vi "Image Display Controller-subvi.vi"() -> ()   [LabVIEW 2014]
doc: "This widget allows the user to separately adjust the properties of mulltiple, independently displayed image windows. The controller is a stand-alone VI that can run in a separate thread from the program that is producing the images, so that the image display settings can be adjusted whilst other things (e.g., data acquisition) are occurring simultaneously."
uses:
  ctt's/Image to Display event.ctt
  <vilib>/vision/Image Controls.llb/IMAQ Image.ctl
  Globals/Initilize Globals.vi
panel:
  in  "Presets":T1(array[cluster])=[{"Mem"=FALSE, "Black"=-32500.0, "White"=-25000.0, "Recall"=FALSE}]
  in  "Keep this in corner?":bool=TRUE
  in  "Autosize M":bool
  in  "Autoposition M":bool
  in  "Autoscale M":bool
  in  "Zoom +":bool
  in  "Zoom -":bool
  out "In use":bool
  in  "Auto size":bool
  in  "Auto position":bool
  in  "Autoscale":bool
  out "Window Title":string
  in  "Control image window #":u8(slide)=1 max=1 step=1 scale=0.0..1.0
  out "error out":errorcluster
  out "Black/White Levels temp":cluster{ext, ext}(slide)={1.0, 65535.0} scale=-32767.0..327567.0
  in  "Black/White Levels":cluster{ext, ext}(slide)={1.0, 65535.0} scale=-32767.0..327567.0
  in  "Stop":bool
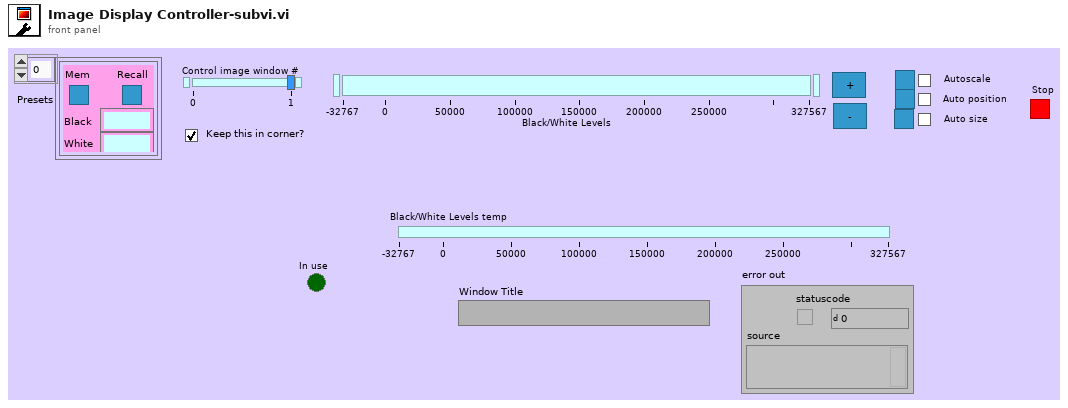
[diagram p1: front panel]
types:
  T1 = cluster{"Mem":bool, "Black":ext, "White":ext, "Recall":bool}[]
  T2 = typedef "Image Type" = u32
  T3 = typedef "IMAQ Image.ctl" = refnum<image>
  T4 = cluster{"Image Type":T2, "Image":T3, "Initialized?":bool, "Window Title":string, "Auto resize?":bool, "Auto position?":bool, "Autoscale?":bool, "Black/White Levels":cluster{ext, ext}, "Scale Min":ext, "Scale Max":ext}
  T5 = typedef "LVRectTypeDef.ctl" = cluster{"Left":i16, "Top":i16, "Right":i16, "Bottom":i16}
  T6 = typedef "Image to Display event.ctt" = cluster{"Image":T3, "Window Title":string, "Window Number":i32, "Image Type":T2, "Quit display controller?":bool}
  T7 = cluster{"Image Type":T2, "Image":T3, "Initialized?":bool, "Window Title":string, "Auto resize?":bool, "Auto position?":bool, "Autoscale?":bool, "Black/White Levels":cluster{ext, ext}, "Scale Min":ext, "Scale Max":ext}[]
  T8 = cluster{"Mem":bool, "Black":ext, "White":ext, "Recall":bool}
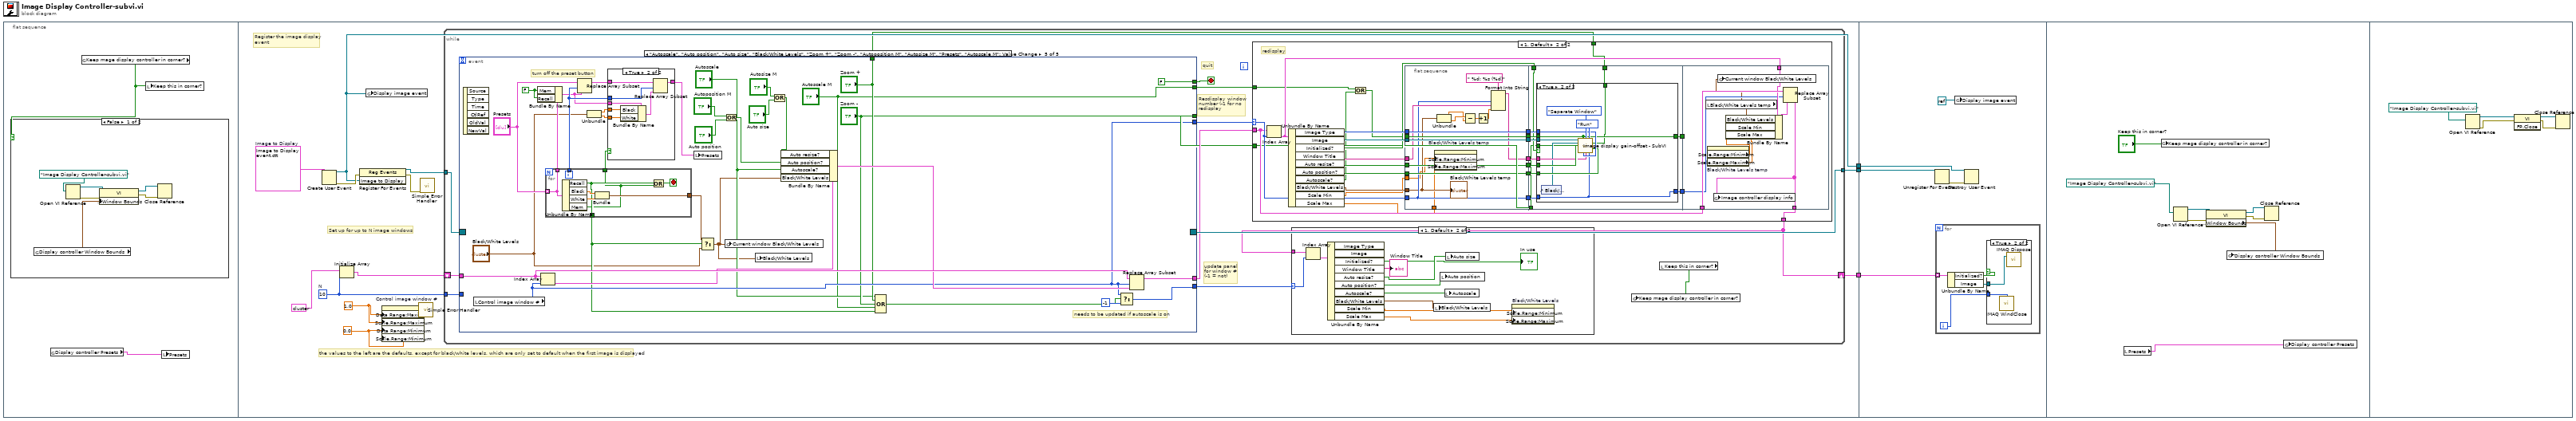
[diagram p0: block diagram]
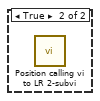
[diagram p2: hidden frame]
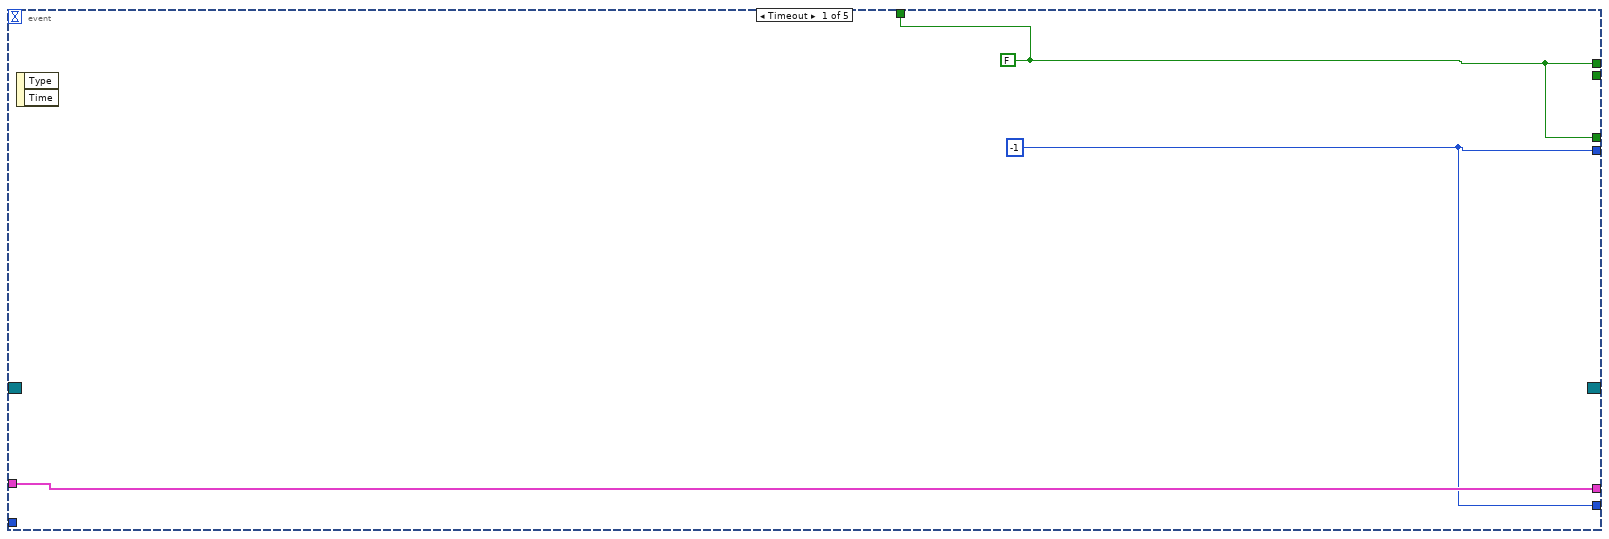
[diagram p6: hidden frame]
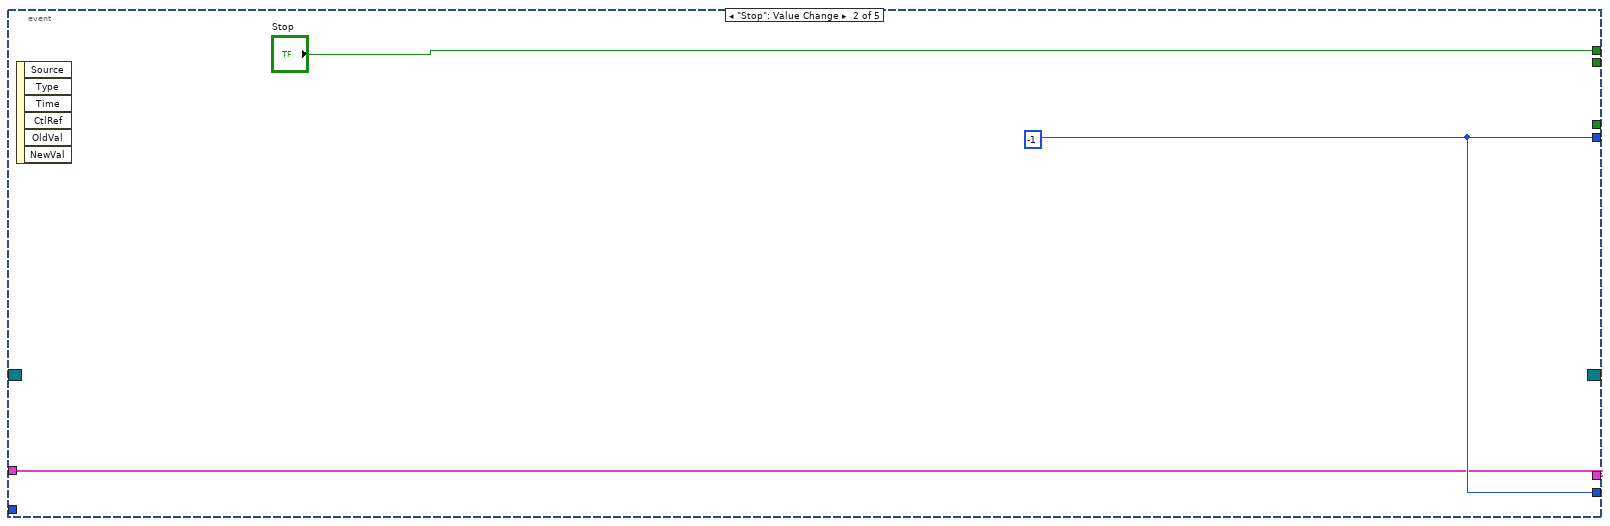
[diagram p7: hidden frame]
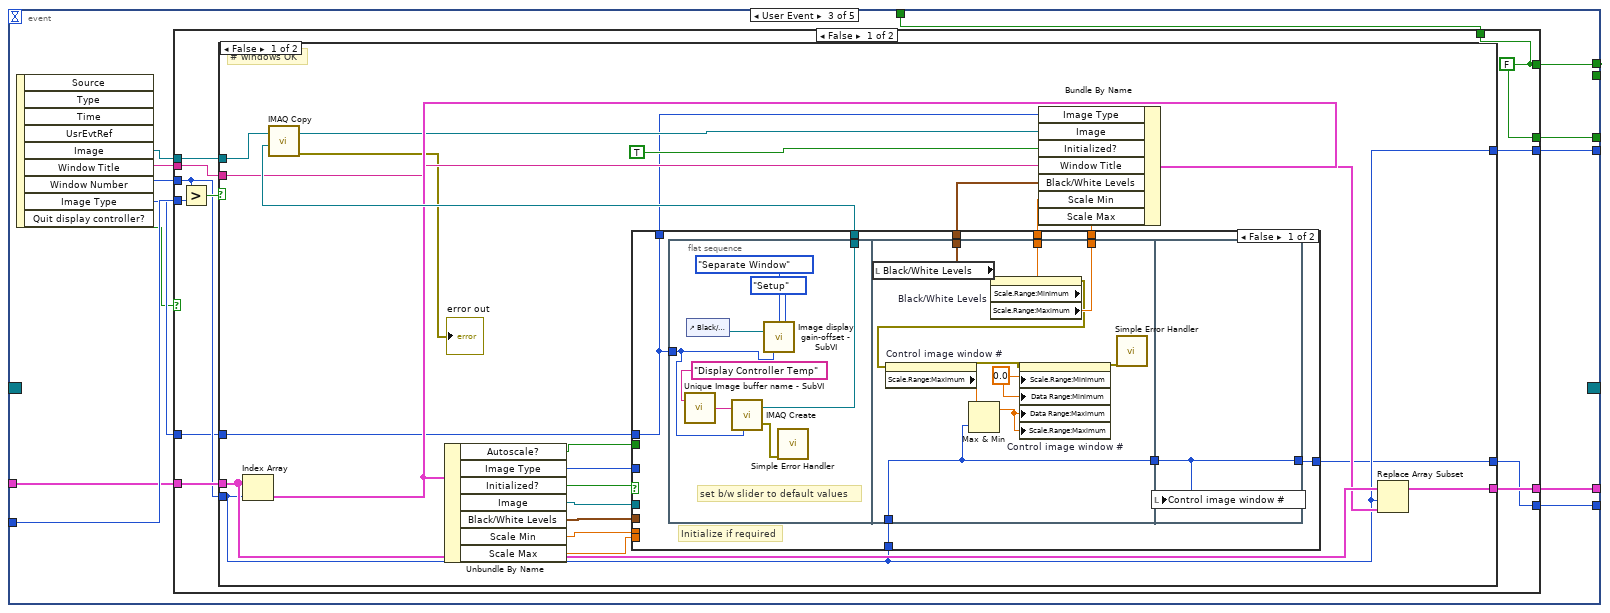
[diagram p8: hidden frame]
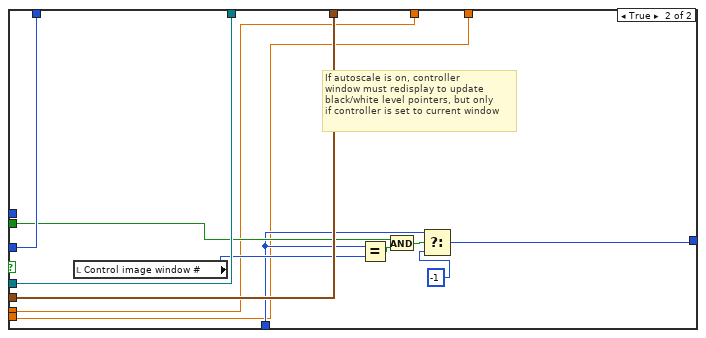
[diagram p9: hidden frame]
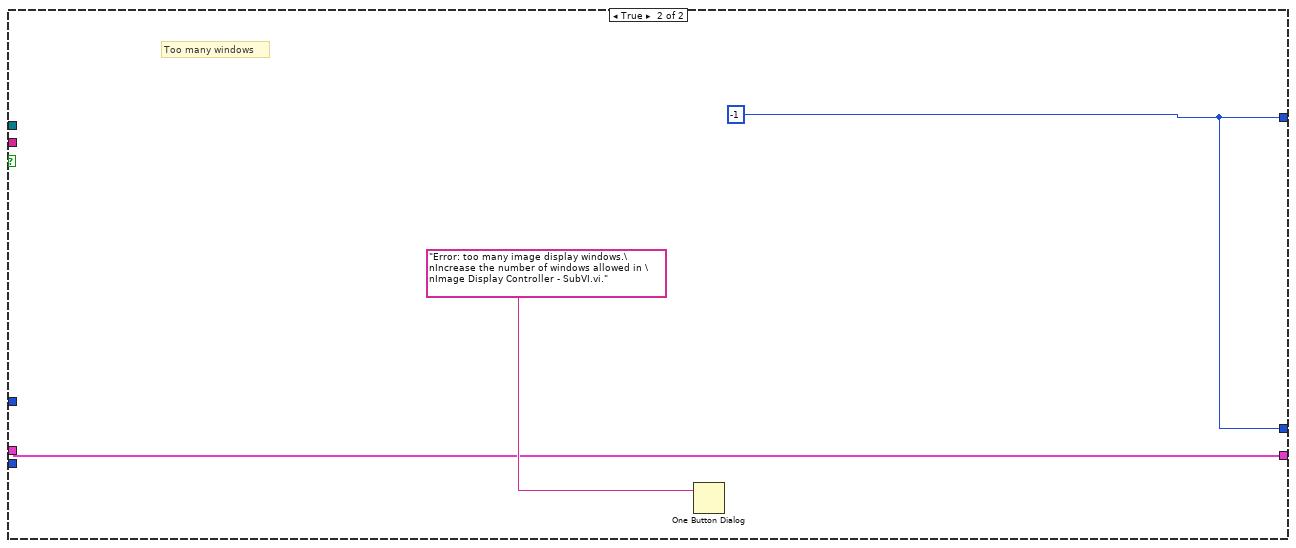
[diagram p10: hidden frame]
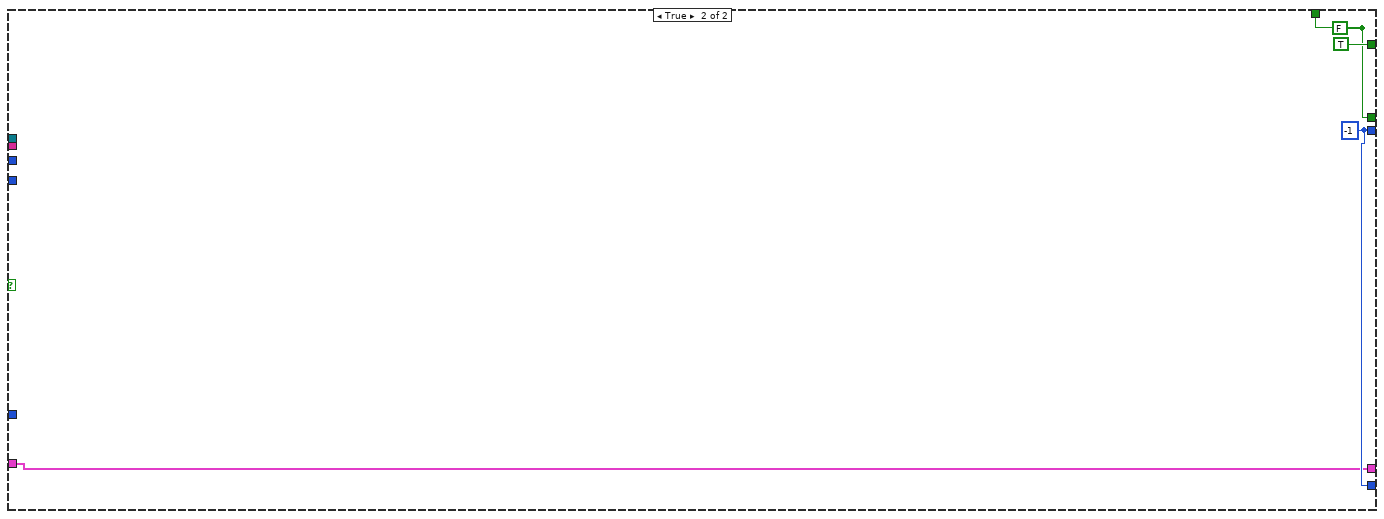
[diagram p11: hidden frame]
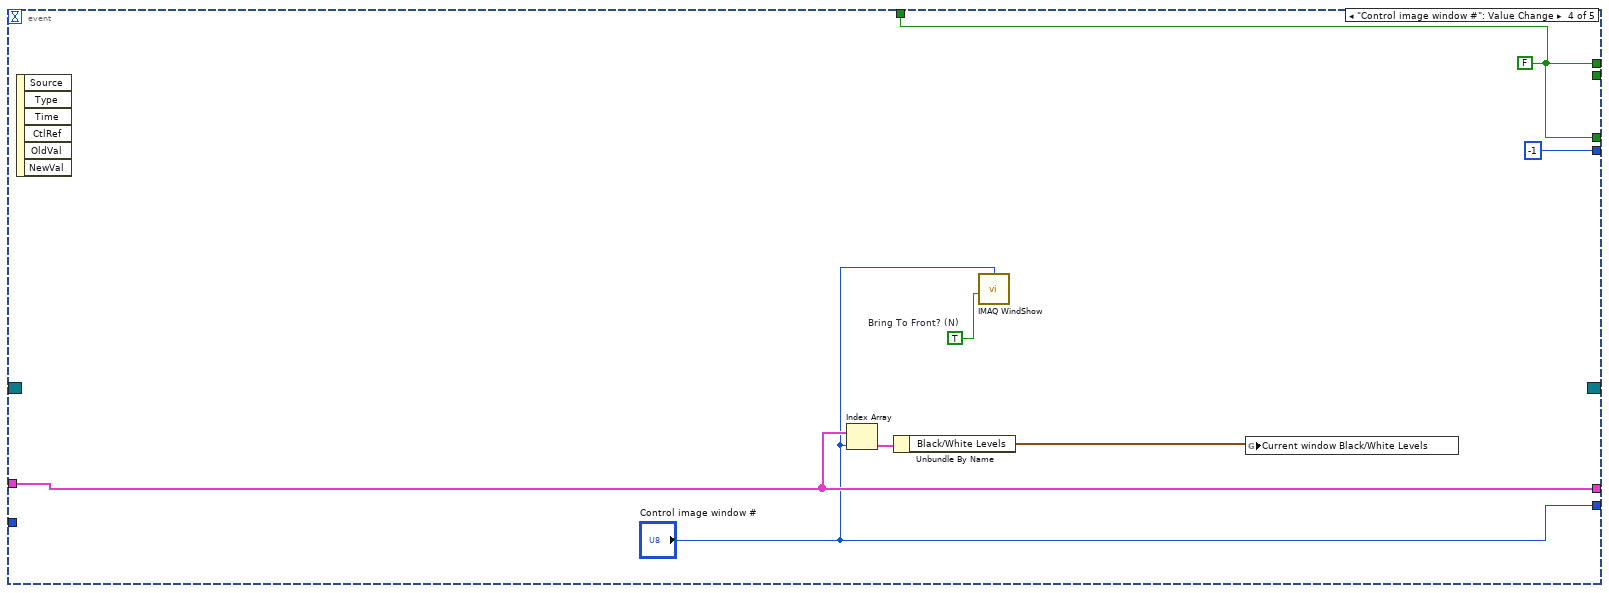
[diagram p12: hidden frame]
diagram:
  n1 = flat-sequence {
    tunnel: [w21] -> w3
    tunnel: [w15] -> w2
    tunnel: [w16] -> w1
    tunnel: w3 -> [w287]
    tunnel: w2 -> [w285]
    tunnel: w1 -> [w283]
    frame #0 {
      n2 = global read "Initilize Globals.vi" "Display controller Presets"() -> (w4:T1)
      n3 = global read "Initilize Globals.vi" "Keep mage display controller in corner?"() -> (w5:bool)
      n4 = case shown="False" w5 {
        frame False {
          n5 = global read "Initilize Globals.vi" "Display controller Window Bounds"() -> (w7:T5)
          n6 = Open VI Reference(vi path=path "Image Display Controller-subvi.vi") -> (vi reference=w11:refnum<vi>, error out=w10:errorcluster)  [unwired: 2 in, 3 out]
          n7 = property class="VI"(reference=w11, error in=w10, "Front Panel Window:Window Bounds"=w7) -> (reference out=w9:refnum<vi>, error out=w8:errorcluster)
          n8 = Close Reference(reference=w9, error in (no error)=w8) -> ()  [unwired: 1 out]
        }
        frame True {
          n9 = call "Position calling vi to LR 2-subvi.vi"() -> ()  [unwired: 4 in, 2 out]
        }
      }
      n10 = local write "Keep this in corner?"(w5) -> ()
      n11 = local write "Presets"(w4) -> ()
    }
    frame #1 {
      w13 = 0.0 ("Data Range:Maximum")
      w14 = 1.0 ("Data Range:Maximum")
      w17 = 10  # N
      w20 = T6 {"Image"=refnum, "Window Title"="", "Window Number"=0, "Image Type"=0, "Quit display controller?"=FALSE}  # Image to Display
      # "the values to the left are the defaults, except for black/white levels, which are only set to default when the first image is displayed"
      # "Set up for up to N image windows"
      # "Register the image display\nevent"
      n12 = Create User Event(user event datatype=w20) -> (user event=w15:refnum<user-event>, error out=w23:errorcluster)  [unwired: 1 in]
      n13 = Initialize Array(T4 {"Image Type"=0, "Image"=refnum, "Initialized?"=FALSE, "Window Title"="", "Auto resize?"=FALSE, "Auto position?"=FALSE, "Autoscale?"=FALSE, "Black/White Levels"={1.0, 2.0}, "Scale Min"=-32767.0, "Scale Max"=327567.0}, w17) -> (w18:T7)
      n14 = register-events(error in=w23, w15) -> (reference out=w24:refnum<event-registration>, error out=w22:errorcluster)  [unwired: 1 in]
      n15 = global write "Initilize Globals.vi" "Display image event"(w15) -> ()
      n16 = property on="Control image window #" class="Slide (strict)"("Data Range:Maximum"=w14, "Scale.Range:Maximum"=w14, "Data Range:Minimum"=w13, "Scale.Range:Minimum"=w13) -> (error out=w12:errorcluster)  [unwired: 2 in, 1 out]
      n17 = call <vilib>:"Simple Error Handler.vi"("error in (no error)"=w12) -> ()  [unwired: 1 in, 8 out]
      n18 = call <vilib>:"Simple Error Handler.vi"("error in (no error)"=w22) -> ()  [unwired: 1 in, 8 out]
      n19 = while {
        shift-right: [w29] -> w16
        shift-left: w18 -> [w35]
        tunnel: w24 -> [w36]
        tunnel: [w32] -> w21
        tunnel: w17 -> [w34]
        stop <- w37 stop-if-true
        # "update panel\nfor window #\n(-1 = not)"
        # "quit"
        # "Resdisplay window\nnumber (-1 for no\nredisplay"
        n20 = event shown="[4] \"Autoscale\", \"Auto position\", \"Auto size\", \"Black/White Levels\", \"Zoom +\", \"Zoom -\", \"Autoposition M\", \"Autosize M\", \"Presets\", \"Autoscale M\": Value Change" {
          selector: w36 -> [_ _ _ _ _]
          dyn-events: [_ _ _ _ _] -> w32
          timeout: _ -> [_ _ _ _ _]
          tunnel: [w127 "Stop" w140 w229 FALSE ("Stop")] -> w37
          tunnel: w35 -> [w129 w130 w144 w232 w266]
          tunnel: w34 -> [_ _ w145 _ _]
          tunnel: [w129 w130 w141 w232 w256] -> w30
          tunnel: [w128 w131 w137 -1 ("Window Number") w260] -> w33
          tunnel: [w128 w131 w136 "Control image window #" w261] -> w31
          tunnel: [w127 _ w133 w229 "Zoom +"] -> w28
          tunnel: [w127 _ w134 w229 "Zoom -"] -> w27
          tunnel: [_ _ _ _ "Autoscale M"] -> w26
          event Timeout {
            w128 = -1 ("Window Number")
            w127 = FALSE ("Stop")
            n21 = event-data() -> ()  [unwired: 3 out]
          }
          event "Stop": Value Change {
            w131 = -1 ("Window Number")
            n22 = event-data() -> ()  [unwired: 7 out]
          }
          event User Event {
            n23 = event-data() -> ("Image"=w138:T3, "Window Title"=w142:string, "Window Number"=w143:i32, "Image Type"=w139:T2, "Quit display controller?"=w135:bool)  [unwired: 5 out]
            n24 = case shown="False" w135 {
              tunnel: w145 -> [w156 _]
              tunnel: w144 -> [w154 w224]
              tunnel: w143 -> [w153 _]
              tunnel: w142 -> [w152 _]
              tunnel: [w151 w224] -> w141
              tunnel: [w146 TRUE] -> w140
              tunnel: w139 -> [w150 _]
              tunnel: w138 -> [w149 _]
              tunnel: [w148 w225] -> w137
              tunnel: [w147 w225] -> w136
              tunnel: [w146 w223] -> w134
              tunnel: [w146 w223] -> w133
              frame False {
                w146 = FALSE
                n25 = Greater?(x=w153, y=w156) -> (0:w155:bool)
                n26 = case shown="False" w155 {
                  tunnel: w154 -> [w171 w221]
                  tunnel: w153 -> [w165 _]
                  tunnel: w149 -> [w177 _]
                  tunnel: w152 -> [w172 _]
                  tunnel: [w157 w221] -> w151
                  tunnel: [w165 w220] -> w148
                  tunnel: w150 -> [w168 _]
                  tunnel: [w164 w220] -> w147
                  frame False {
                    # "# windows OK"
                    n27 = Index Array(array=w171, index=w165) -> (element=w176:T4)
                    n28 = Unbundle By Name(w176) -> ("Autoscale?"=w162:bool, "Image Type"=w173:T2, "Initialized?"=w180:bool, "Image"=w179:T3, "Black/White Levels"=w166:cluster{ext, ext}, "Scale Min"=w159:ext, "Scale Max"=w158:ext)
                    n29 = case shown="False" w180 {
                      tunnel: w173 -> [_ w218]
                      tunnel: [w188 w219] -> w178
                      tunnel: w179 -> [_ w219]
                      tunnel: [w187 w218] -> w169
                      tunnel: w168 -> [w187 _]
                      tunnel: w166 -> [_ w217]
                      tunnel: [w186 w217] -> w163
                      tunnel: w165 -> [w185 w210]
                      tunnel: [w184 w214] -> w164
                      tunnel: w162 -> [_ w215]
                      tunnel: [w183 w209] -> w161
                      tunnel: [w182 w208] -> w160
                      tunnel: w159 -> [_ w209]
                      tunnel: w158 -> [_ w208]
                      frame False {
                        # "Initialize if required"
                        n30 = flat-sequence {
                          tunnel: [w194] -> w188
                          tunnel: w187 -> [w189]
                          tunnel: [w206] -> w186
                          tunnel: w185 -> [w201]
                          tunnel: [w204] -> w183
                          tunnel: [w203] -> w182
                          tunnel: [w201] -> w181
                          tunnel: [w207] -> w184
                          tunnel: w181 -> [w207]
                          frame #0 {
                            # "set b/w slider to default values"
                            n31 = call "Unique Image buffer name - SubVI.vi"("Buffer  base name"="Display Controller Temp") -> ("Image Name"=w195:string)  [unwired: 1 in]
                            n32 = control-ref of="Black/White Levels"() -> (w190:refnum<vi>)
                            n33 = call "IMAQ Create"("Image Name"=w195, "Image Type"=w189) -> ("New Image"=w194:T3, "error out"=w193:errorcluster)  [unwired: 2 in, 1 out]
                            n34 = call "Image display gain-offset - SubVI.vi"("Display Type (s)"=enum16{"Front Panel", "Separate Window"}."Separate Window", "Mode"=enum16{"Setup", "Run"}."Setup", "Black/White Levels Ctl Ref (s)"=w190, "Pixel depth (s)"=w189) -> ()  [unwired: 10 in, 2 out]
                            n35 = call <vilib>:"Simple Error Handler.vi"("error in (no error)"=w193) -> ()  [unwired: 1 in, 8 out]
                          }
                          frame #1 {
                            w205 = 0.0 ("Data Range:Minimum")
                            n36 = local read "Black/White Levels"() -> (w206:cluster{ext, ext})
                            n37 = property on="Black/White Levels" class="Slide (strict)"() -> (error out=w199:errorcluster, "Scale.Range:Minimum"=w204:dbl, "Scale.Range:Maximum"=w203:dbl)  [unwired: 2 in, 1 out]
                            n38 = property on="Control image window #" class="Slide (strict)"(error in=w199) -> (error out=w198:errorcluster, "Scale.Range:Maximum"=w202:dbl)  [unwired: 1 in, 1 out]
                            n39 = Max & Min(x=w202, y=w201) -> (max(x,y)=w200:dbl)  [unwired: 1 out]
                            n40 = property on="Control image window #" class="Slide (strict)"(error in=w198, "Scale.Range:Minimum"=w205, "Data Range:Minimum"=w205, "Data Range:Maximum"=w200, "Scale.Range:Maximum"=w200) -> (error out=w197:errorcluster)  [unwired: 1 in, 1 out]
                            n41 = call <vilib>:"Simple Error Handler.vi"("error in (no error)"=w197) -> ()  [unwired: 1 in, 8 out]
                          }
                          frame #2 {
                            n42 = local write "Control image window #"(w207) -> ()
                          }
                        }
                      }
                      frame True {
                        # "If autoscale is on, controller\nwindow must redisplay to update \nblack/white level pointers, but only\nif controller is set to current window"
                        n43 = local read "Control image window #"() -> (w211:u8)
                        n44 = Equal?(x=w210, y=w211) -> (x = y?=w212:bool)
                        n45 = And(x=w215, y=w212) -> (x .and. y?=w213:bool)
                        n46 = Select(t=w210, s=w213, f=-1 ("Window Number")) -> (s? t:f=w214:i32)
                      }
                    }
                    n47 = call "IMAQ Copy"("Image Dst"=w178, "Image Src"=w177) -> ("error out"=→"error out":errorcluster, "Image Dst Out"=w175:T3)  [unwired: 1 in, 3 out]
                    n48 = Bundle By Name(cluster=w176, "Image Type"=w169, "Image"=w175, "Initialized?"=TRUE, "Window Title"=w172, "Black/White Levels"=w163, "Scale Min"=w161, "Scale Max"=w160) -> (w170:T4)
                    n49 = Replace Array Subset(array=w171, new element=w170, index=w165) -> (w157:T7)
                  }
                  frame True {
                    w220 = -1 ("Window Number")
                    # "Too many windows"
                    n50 = One Button Dialog(message="Error: too many image display windows.\nIncrease the number of windows allowed in \nImage Display Controller - SubVI.vi.") -> ()  [unwired: 2 out]
                  }
                }
              }
              frame True {
                w223 = FALSE
                w225 = -1 ("Window Number")
              }
            }
          }
          event "Control image window #": Value Change {
            w228 = TRUE  # Bring To Front? (N)
            w229 = FALSE ("Stop")
            n51 = event-data() -> ()  [unwired: 7 out]
            n52 = Index Array(array=w232, index="Control image window #") -> (element=w231:T4)
            n53 = Unbundle By Name(w231) -> ("Black/White Levels"=w230:cluster{ext, ext})
            n54 = call "IMAQ WindShow"("Bring To Front? (N)"=w228, "Window Number (0...15)"="Control image window #") -> ()  [unwired: 3 in, 4 out]
            n55 = global write "Initilize Globals.vi" "Current window Black/White Levels"(w230) -> ()
          }
          event "Autoscale", "Auto position", "Auto size", "Black/White Levels", "Zoom +", "Zoom -", "Autoposition M", "Autosize M", "Presets", "Autoscale M": Value Change {
            w243 = FALSE ("Select")
            # "turn off the preset button"
            # "needs to be updated if autoscale is on"
            n56 = event-data() -> ()  [unwired: 7 out]
            n57 = local read "Control image window #"() -> (w260:u8)
            n58 = Index Array(array=w266, index=w260) -> (element=w265:T4)
            n59 = for {
              tunnel: "Presets" -> [w278] mode=indexing
              tunnel: [w280] -> w247
              tunnel: [w276] -> w244
              tunnel: [w279] -> w240
              tunnel: [w278] -> w246
              tunnel: [w275] -> w239
              i -> [w279]
              stop <- w277 stop-if-true
              n60 = Unbundle By Name(w278) -> ("Recall"=w276:bool, "Black"=w282:ext, "White"=w281:ext, "Mem"=w275:bool)
              n61 = Bundle("Black"=w282, "White"=w281) -> (w280:cluster{"Black":ext, "White":ext})  [unwired: 1 out]
              n62 = Or(x=w276, y=w275) -> (x .or. y?=w277:bool)
            }
            n63 = Bundle By Name(cluster=w246, "Mem"=w243, "Recall"=w243) -> (w238:T8)
            n64 = Replace Array Subset(array="Presets", new element=w238, index=w240) -> (w242:T1)
            n65 = Unbundle("Black/White Levels") -> (w235:ext, w236:ext)
            n66 = case shown="True" w239 {
              tunnel: w242 -> [w267 w274]
              tunnel: [w267 w273] -> w241
              tunnel: w240 -> [_ w272]
              tunnel: w238 -> [_ w271]
              tunnel: w236 -> [_ w269]
              tunnel: w235 -> [_ w268]
              frame False {
              }
              frame True {
                n67 = Bundle By Name(cluster=w271, "Black"=w268, "White"=w269) -> (w270:T8)
                n68 = Replace Array Subset(array=w274, new element=w270, index=w272) -> (w273:T1)
              }
            }
            n69 = local write "Presets"(w241) -> ()
            n70 = Select(t=w247, s=w244, f="Black/White Levels") -> (s? t:f=w234:cluster{"Black":ext, "White":ext})
            n71 = Or(x="Autoposition M", y="Auto position") -> (x .or. y?=w254:bool)
            n72 = global write "Initilize Globals.vi" "Current window Black/White Levels"(w234) -> ()
            n73 = local write "Black/White Levels"(w234) -> ()
            n74 = Or(x="Autosize M", y="Auto size") -> (x .or. y?=w252:bool)
            n75 = Bundle By Name(cluster=w265, "Auto resize?"=w252, "Auto position?"=w254, "Autoscale?"="Autoscale", "Black/White Levels"=w234) -> (w264:T4)
            n76 = Compound Arithmetic op=OR("Autoscale", "Zoom +", "Zoom -", "Autoscale M", w244) -> (w259:bool)
            n77 = Select(t=w260, s=w259, f=-1) -> (s? t:f=w261:i32)
            n78 = Replace Array Subset(array=w266, new element=w264, index=w260) -> (w256:T7)
          }
        }
        n79 = case shown="1, Default" w33 {
          selector: w33 -> [_ w73]
          tunnel: w30 -> [w49 w61]
          tunnel: [w49 w58] -> w29
          tunnel: w28 -> [_ w54]
          tunnel: w27 -> [_ w53]
          tunnel: w26 -> [_ w50]
          frame -1 {
          }
          frame 1, Default {
            # "redisplay"
            n80 = Index Array(array=w61, index=w73) -> (element=w59:T4)
            n81 = Unbundle By Name(w59) -> ("Image Type"=w74:T2, "Image"=w76:T3, "Initialized?"=w62:bool, "Window Title"=w72:string, "Auto resize?"=w75:bool, "Auto position?"=w71:bool, "Autoscale?"=w51:bool, "Black/White Levels"=w63:cluster{ext, ext}, "Scale Min"=w56:ext, "Scale Max"=w55:ext)
            n82 = Or(x=w50, y=w51) -> (x .or. y?=w52:bool)
            n83 = flat-sequence {
              tunnel: w71 -> [w88]
              tunnel: w72 -> [w86]
              tunnel: w73 -> [w84]
              tunnel: w74 -> [w89]
              tunnel: w75 -> [w90]
              tunnel: w76 -> [w91]
              tunnel: w52 -> [w92]
              tunnel: [w92] -> w70
              tunnel: [w91] -> w69
              tunnel: [w90] -> w68
              tunnel: [w89] -> w67
              tunnel: [w84] -> w66
              tunnel: [w85] -> w65
              tunnel: [w88] -> w64
              tunnel: w63 -> [w83]
              tunnel: w56 -> [w78]
              tunnel: w55 -> [w77]
              tunnel: w70 -> [w104]
              tunnel: w69 -> [w103]
              tunnel: w68 -> [w102]
              tunnel: w67 -> [w101]
              tunnel: w66 -> [w100]
              tunnel: w65 -> [w99]
              tunnel: w64 -> [w98]
              tunnel: w62 -> [w97]
              tunnel: [w96] -> w60
              tunnel: [w95] -> w57
              tunnel: w54 -> [w94]
              tunnel: w53 -> [w93]
              tunnel: w61 -> [w126]
              tunnel: w60 -> [w124]
              tunnel: w59 -> [w125]
              tunnel: [w120] -> w58
              tunnel: w57 -> [_]
              frame #0 {
                n84 = property on="Black/White Levels temp" class="Slide (strict)"("Scale.Range:Minimum"=w78, "Scale.Range:Maximum"=w77) -> ()  [unwired: 2 in, 2 out]
                n85 = Unbundle(w83) -> (w81:ext, w82:ext)
                n86 = Subtract(x=w82, y=w81) -> (x-y=w80:ext)
                n87 = Increment(x=w80) -> (x+1=w79:ext)
                n88 = Format Into String(format string=" %d: %s (%d)", w84, w86, w79) -> (resulting string=w85:string)  [unwired: 2 in, 1 out]
                "Black/White Levels temp" <- w83
              }
              frame #1 {
                n89 = case shown="True" w97 {
                  tunnel: w104 -> [w105 w110]
                  tunnel: w103 -> [_ w116]
                  tunnel: w102 -> [_ w115]
                  tunnel: w101 -> [_ w114]
                  tunnel: w100 -> [w106 w107]
                  tunnel: w99 -> [_ w113]
                  tunnel: w98 -> [_ w112]
                  tunnel: [w106 w107] -> w96
                  tunnel: [w105 w110] -> w95
                  tunnel: w94 -> [_ w109]
                  tunnel: w93 -> [_ w108]
                  frame False {
                  }
                  frame True {
                    n90 = control-ref of="Black/White Levels temp"() -> (w111:refnum<vi>)
                    n91 = call "Image display gain-offset - SubVI.vi"("Image In"=w116, "Autoscale?"=w110, "Display Type (s)"=enum16{"Front Panel", "Separate Window"}."Separate Window", "Mode"=enum16{"Setup", "Run"}."Run", "Black/White Levels Ctl Ref (s)"=w111, "Zoom +"=w109, "Auto Resize to Image Size?\n(Window only)"=w115, "Zoom -"=w108, "Auto position\n(Window only)"=w112, "Pixel depth (s)"=w114, "Window Title\n(Window only)"=w113, "Window Number\n(Window only)"=w107) -> ()  [unwired: 2 in, 2 out]
                  }
                }
              }
              frame #2 {
                n92 = local read "Black/White Levels temp"() -> (w119:cluster{ext, ext})
                n93 = property on="Black/White Levels temp" class="Slide (strict)"() -> ("Scale.Range:Minimum"=w122:dbl, "Scale.Range:Maximum"=w121:dbl)  [unwired: 2 in, 2 out]
                n94 = global write "Initilize Globals.vi" "Current window Black/White Levels"(w119) -> ()
                n95 = Bundle By Name(cluster=w125, "Black/White Levels"=w119, "Scale Min"=w122, "Scale Max"=w121) -> (w123:T4)
                n96 = Replace Array Subset(array=w126, new element=w123, index=w124) -> (w120:T7)
                n97 = global write "Initilize Globals.vi" "Image controller display info"(w120) -> ()
              }
            }
          }
        }
        n98 = case shown="1, Default" w31 {
          selector: w31 -> [_ w41]
          tunnel: w29 -> [_ w47]
          frame -1 {
          }
          frame 1, Default {
            n99 = Index Array(array=w47, index=w41) -> (element=w48:T4)
            n100 = Unbundle By Name(w48) -> ("Initialized?"=→"In use":bool, "Window Title"=→"Window Title":string, "Auto resize?"=w44:bool, "Auto position?"=w43:bool, "Autoscale?"=w42:bool, "Black/White Levels"=w45:cluster{ext, ext}, "Scale Min"=w38:ext, "Scale Max"=w39:ext)  [unwired: 2 out]
            n101 = local write "Black/White Levels"(w45) -> ()
            n102 = local write "Auto position"(w43) -> ()
            n103 = local write "Autoscale"(w42) -> ()
            n104 = local write "Auto size"(w44) -> ()
            n105 = property on="Black/White Levels" class="Slide (strict)"("Scale.Range:Minimum"=w38, "Scale.Range:Maximum"=w39) -> ()  [unwired: 2 in, 2 out]
          }
        }
        n106 = local read "Keep this in corner?"() -> (w25:bool)
        n107 = global write "Initilize Globals.vi" "Keep mage display controller in corner?"(w25) -> ()
      }
    }
    frame #2 {
      n108 = Unregister For Events(event registration refnum=w287) -> (error out=w286:errorcluster)  [unwired: 1 in]
      n109 = for {
        tunnel: w283 -> [w291] mode=indexing
        i -> [w288]
        n110 = Unbundle By Name(w291) -> ("Initialized?"=w290:bool, "Image"=w289:T3)
        n111 = case shown="True" w290 {
          tunnel: w289 -> [_ w293]
          tunnel: w288 -> [_ w292]
          frame False {
          }
          frame True {
            n112 = call "IMAQ WindClose"("Window Number (0...15)"=w292) -> ()  [unwired: 2 in, 4 out]
            n113 = call "IMAQ Dispose"("Image"=w293) -> ()  [unwired: 2 in, 4 out]
          }
        }
      }
      n114 = global write "Initilize Globals.vi" "Display image event"(refnum<k0> refnum) -> ()
      n115 = Destroy User Event(user event=w285, error in=w286) -> ()  [unwired: 1 out]
    }
    frame #3 {
      n116 = local read "Presets"() -> (w294:T1)
      n117 = global write "Initilize Globals.vi" "Keep mage display controller in corner?"("Keep this in corner?") -> ()
      n118 = Open VI Reference(vi path=path "Image Display Controller-subvi.vi") -> (vi reference=w300:refnum<vi>, error out=w299:errorcluster)  [unwired: 1 in, 4 out]
      n119 = property class="VI"(reference=w300, error in=w299) -> (reference out=w298:refnum<vi>, error out=w297:errorcluster, "Front Panel Window:Window Bounds"=w296:T5)
      n120 = global write "Initilize Globals.vi" "Display controller Window Bounds"(w296) -> ()
      n121 = Close Reference(reference=w298, error in (no error)=w297) -> ()  [unwired: 1 out]
      n122 = global write "Initilize Globals.vi" "Display controller Presets"(w294) -> ()
    }
    frame #4 {
      n123 = Open VI Reference(vi path=path "Image Display Controller-subvi.vi") -> (vi reference=w303:refnum<vi>, error out=w304:errorcluster)  [unwired: 1 in, 4 out]
      n124 = invoke class="VI" method="FP.Close"(reference=w303, error in=w304) -> (reference out=w305:refnum<vi>, error out=w306:errorcluster)  [unwired: 1 in, 1 out]
      n125 = Close Reference(reference=w305, error in (no error)=w306) -> ()  [unwired: 1 out]
    }
  }
